vi "AB_860_900_Project_WebService_Info.vi"(7 "action":T2, 8 "error in (no error)":errorcluster, 10 "webServiceInfo in":T1, 11 "Object In":T3) -> (0 "error out":errorcluster, 2 "webServiceInfo out":T1, 3 "Object Out":T3)   [LabVIEW 2020]
uses:
  <resource>/Framework/Providers/API/ItemRef.ctl
  <vilib>/AppBuilder/RW_Project/AB_RW_Project_PropBag_Action.ctl
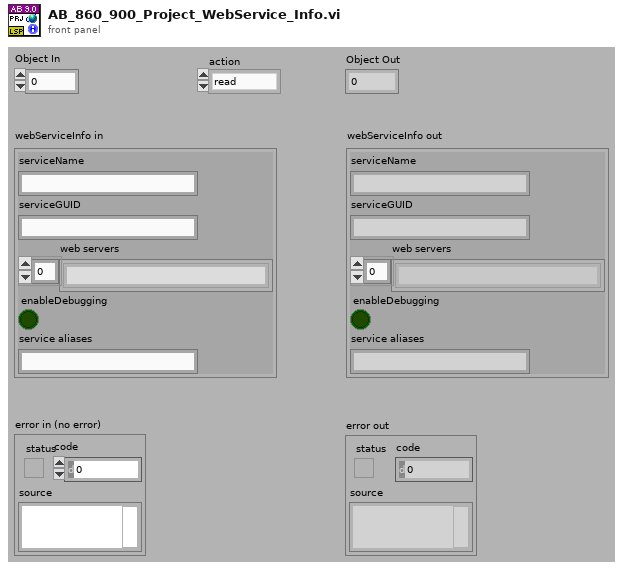
[diagram p1: front panel]
types:
  T1 = cluster{"serviceName":string, "serviceGUID":string, "web servers":string[], "enableDebugging":bool, "service aliases":string}
  T2 = typedef "AB_RW_Project_PropBag_Action.ctl" = enum16{"read", "write", "clear", "readPrevious", "writePrevious", "clearPrevious"}
  T3 = typedef "ItemRef.ctl" = u64
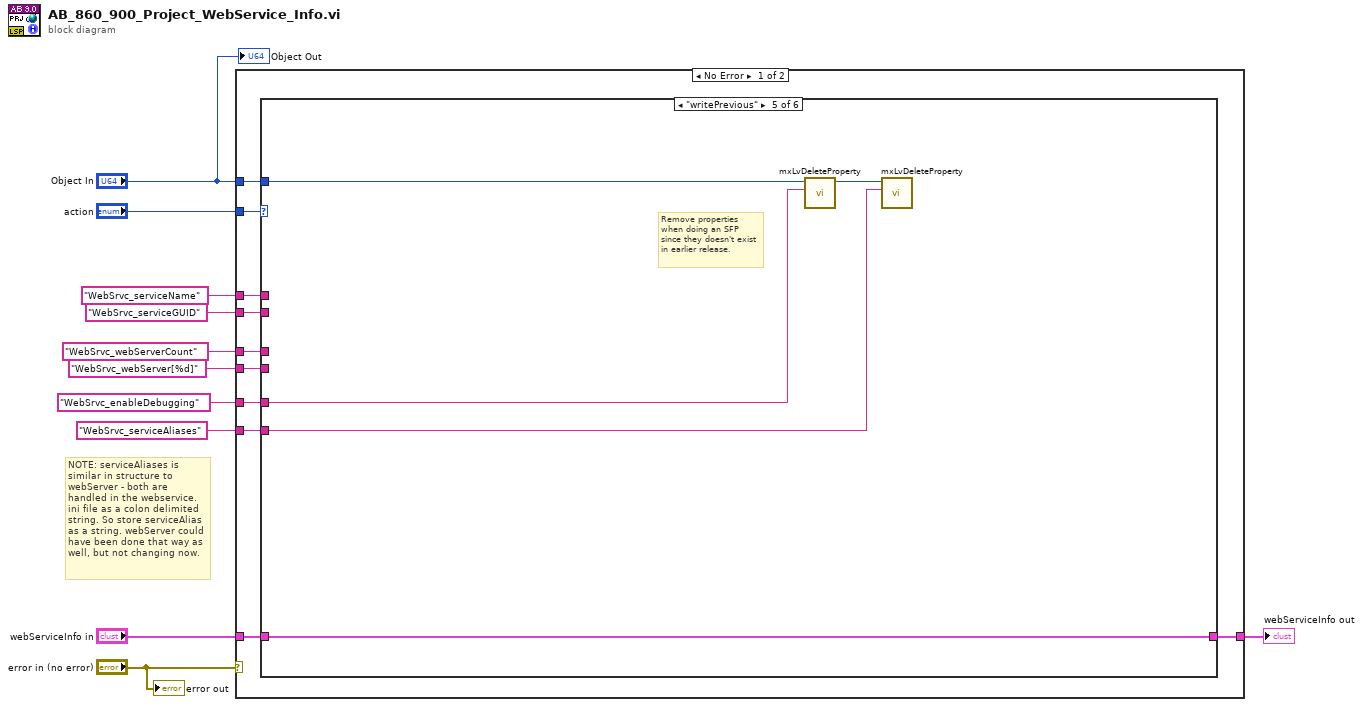
[diagram p0: block diagram]
diagram:
  # "NOTE: serviceAliases is similar in structure to webServer - both are handled in the webservice.ini file as a colon delimited string. So store serviceAlias as a string. webServer could have been done that way as well, but not changing now."
  n1 = case shown="No Error" "error in (no error)" {
    tunnel: "Object In" -> [w21 _]
    tunnel: [w15 _] -> w3
    tunnel: "WebSrvc_serviceGUID" ("Tag") -> [w20 _]
    tunnel: "WebSrvc_webServerCount" ("Tag") -> [w19 _]
    tunnel: "WebSrvc_webServer[%d]" ("Tag") -> [w18 _]
    tunnel: "webServiceInfo in" -> [w17 _]
    tunnel: "action" -> [w16 _]
    tunnel: "WebSrvc_serviceName" ("Tag") -> [w14 _]
    tunnel: "WebSrvc_enableDebugging" ("Tag") -> [w13 _]
    tunnel: "WebSrvc_serviceAliases" ("Tag") -> [w12 _]
    frame No Error {
      n2 = case shown="\"writePrevious\"" w16 {
        tunnel: w21 -> [_ _ _ _ w29 _]
        tunnel: w20 -> [_ _ _ _ _ _]
        tunnel: w19 -> [_ _ _ _ _ _]
        tunnel: w18 -> [_ _ _ _ _ _]
        tunnel: w17 -> [w22 w23 w24 w25 w30 w31]
        tunnel: [w22 w23 w24 w25 w30 w31] -> w15
        tunnel: w14 -> [_ _ _ _ _ _]
        tunnel: w13 -> [_ _ _ _ w28 _]
        tunnel: w12 -> [_ _ _ _ w26 _]
        frame "read" {
        }
        frame "write" {
        }
        frame "clear" {
        }
        frame "readPrevious" {
        }
        frame "writePrevious" {
          # "Remove properties when doing an SFP since they doesn't exist in earlier release."
          n3 = call <resource>:"mxLvDeleteProperty.vi"("Tag"=w28, "Item"=w29) -> ("Item"=w27:T3)  [unwired: 1 in, 8 out]
          n4 = call <resource>:"mxLvDeleteProperty.vi"("Tag"=w26, "Item"=w27) -> ()  [unwired: 1 in, 9 out]
        }
        frame "clearPrevious" {
        }
      }
    }
    frame Error {
    }
  }
  "webServiceInfo out" <- w3
  "Object Out" <- "Object In"
  "error out" <- "error in (no error)"
